vi "ai_continuous_and_ao_waveform_pc_infinite.vi"() -> ()   [LabVIEW 2020]
uses:
  <vilib>/measure/NI_MABase.lvlib
panel:
  out "error out 2":errorcluster caption="错误输出"
  in  "停止":bool
  out "Rounds 2":i32
  out "x-y":u32
  out "波形图 2":waveform(dbl)(graph)
  in  "SamplePeriod":u32=10000
  in  "Chan":u8
  out "Rounds":i32
  out "error out":errorcluster caption="错误输出"
  out "AiFifoResidual":i32
  in  "Stop":bool
  out "波形图":sgl[][](graph)
  in  "PointsToRead":u32=500
  in  "SamplePeriod(ns)":u32=20000
  in  "ChanSel":bool[](array[boolean])=[TRUE, TRUE, TRUE, TRUE, TRUE, TRUE, TRUE, TRUE, FALSE, FALSE, FALSE, FALSE, FALSE, FALSE, FALSE, FALSE, FALSE, FALSE, FALSE, FALSE, FALSE, FALSE, FALSE, FALSE]
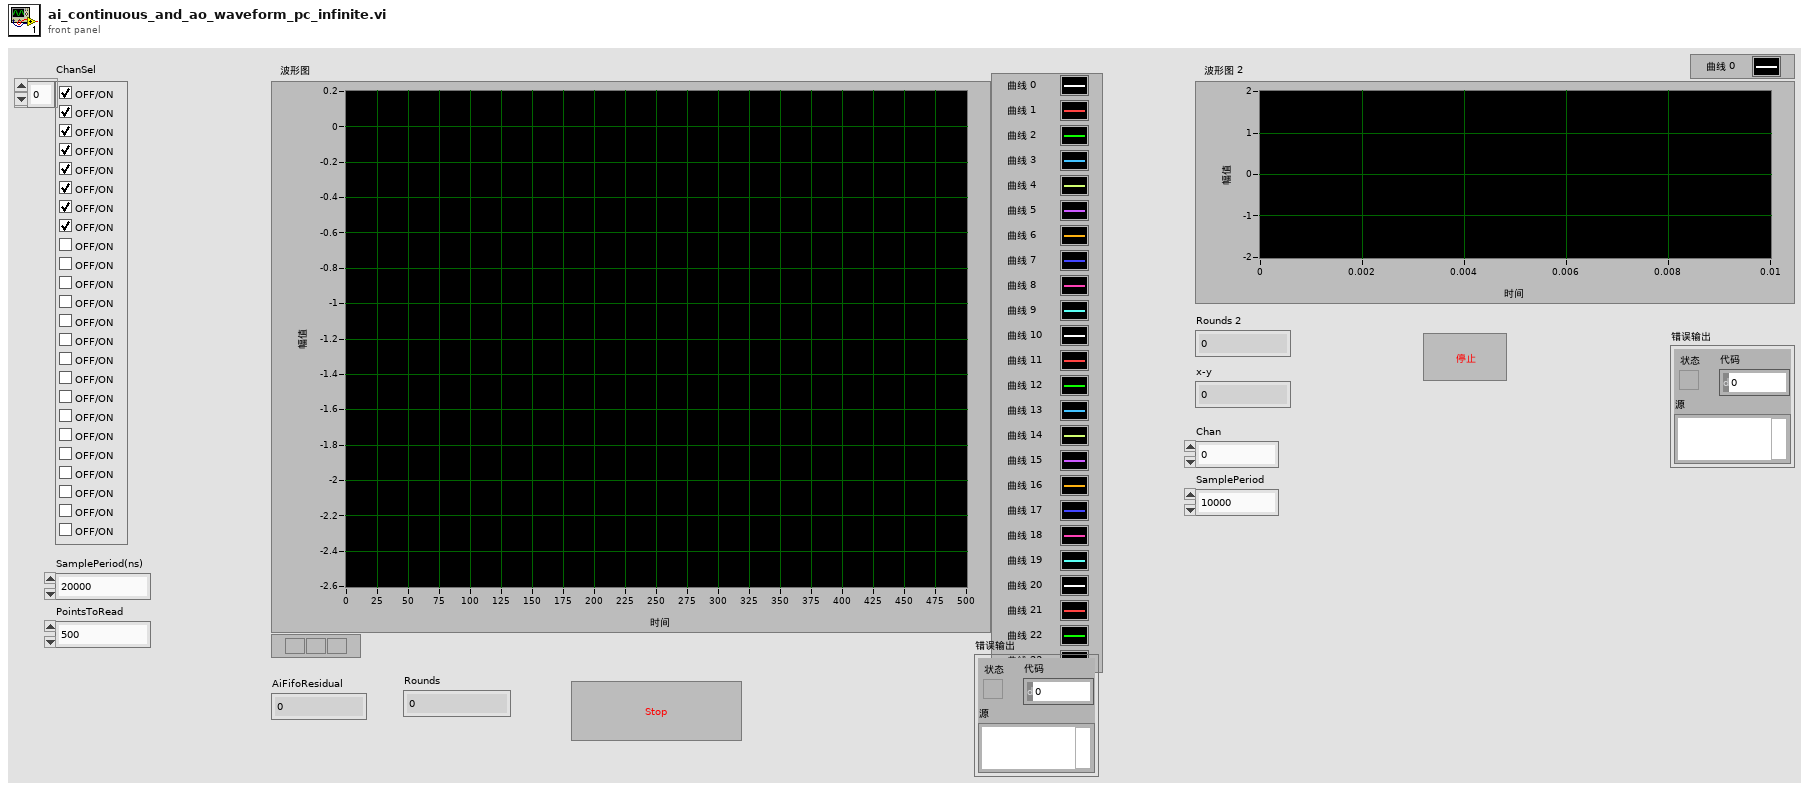
[diagram p1: front panel]
types:
  T1 = enum16{"Sine Wave", "Triangle Wave", "Square Wave", "Sawtooth Wave"}
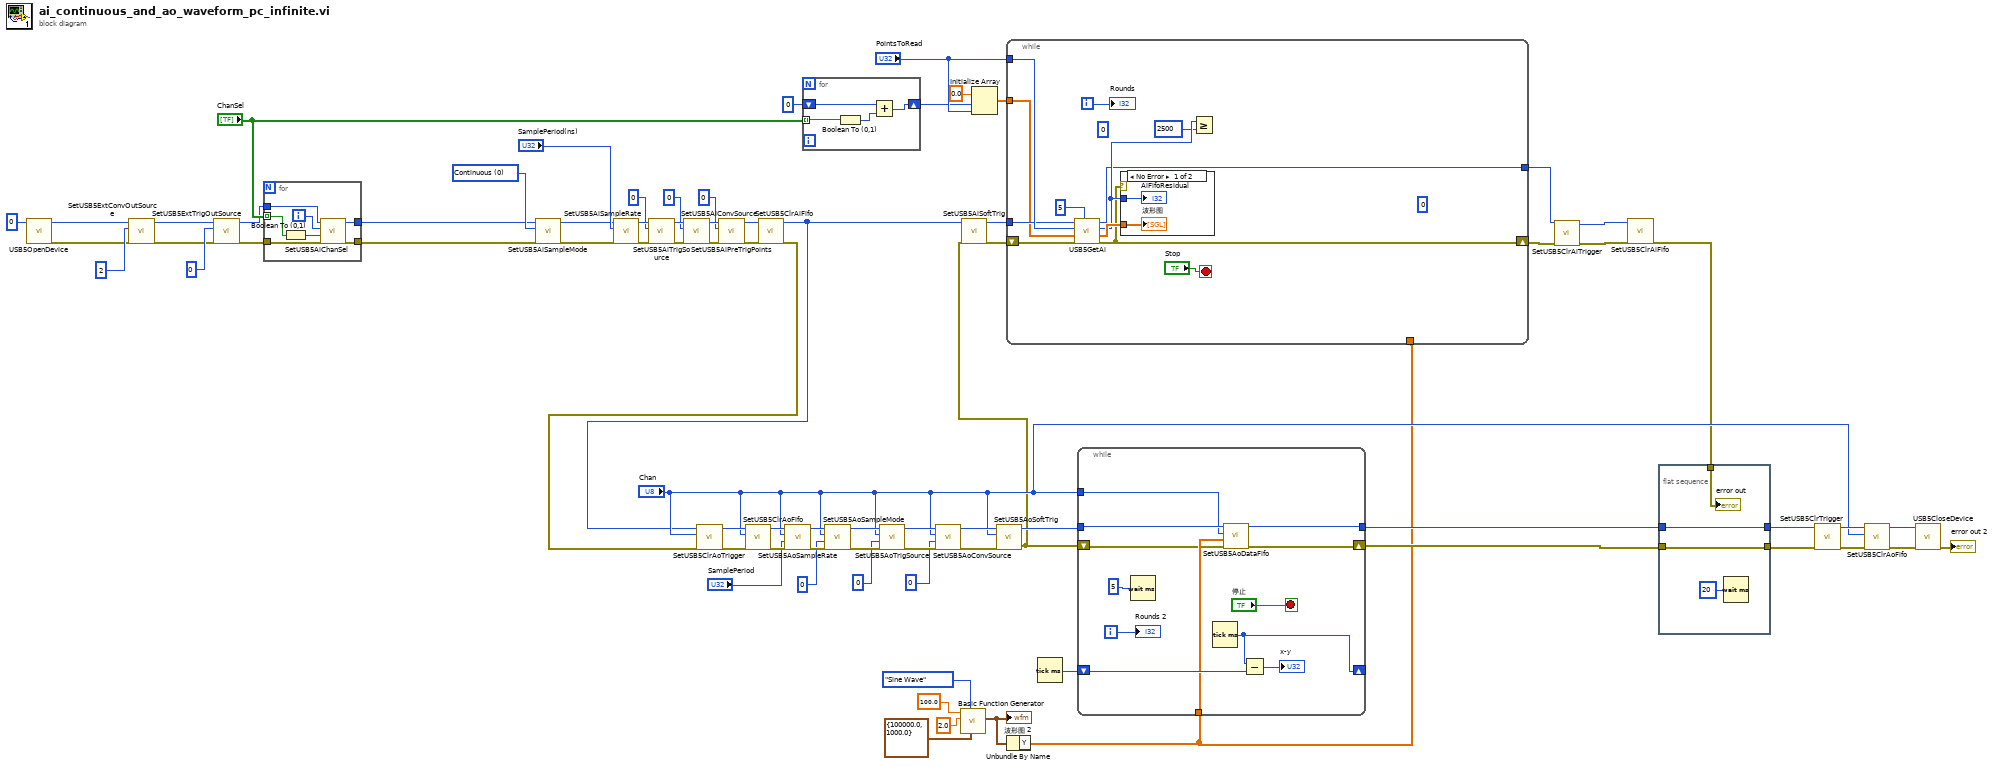
[diagram p0: block diagram]
diagram:
  w74 = u8 0 items=["Continuous", "OneShot"] ("AiSampleMode")
  n1 = call "USB5OpenDevice.vi"("DevIndex"=0) -> ("error out"=w48:errorcluster, "DevIndex Out"=w49:i32)  [unwired: 9 in]
  n2 = call "SetUSB5ExtConvOutSource.vi"("错误输入（无错误）"=w48, "Source"=u8 2, "DevIndex"=w49) -> ("错误输出"=w46:errorcluster, "DevIndex Out"=w47:i32)  [unwired: 7 in]
  n3 = call "SetUSB5ExtTrigOutSource.vi"("错误输入（无错误）"=w46, "Source"=u8 0, "DevIndex"=w47) -> ("错误输出"=w50:errorcluster, "DevIndex Out"=w51:i32)  [unwired: 7 in]
  n4 = for {
    tunnel: w51 -> [w83]
    tunnel: w50 -> [w82]
    tunnel: [w79] -> w4
    tunnel: [w78] -> w3
    tunnel: "ChanSel" -> [w77] mode=indexing
    i -> [w81]
    n5 = Boolean To (0,1)(Boolean=w77) -> (0, 1=w80:i16)
    n6 = call "SetUSB5AiChanSel.vi"("错误输入（无错误）"=w82, "Sel"=w80, "Chan"=w81, "DevIndex"=w83) -> ("错误输出"=w78:errorcluster, "DevIndex Out"=w79:i32)  [unwired: 6 in]
  }
  n7 = call "SetUSB5AiSampleMode.vi"("错误输入（无错误）"=w3, "AiSampleMode"=w74, "DevIndex"=w4) -> ("错误输出"=w5:errorcluster, "DevIndex Out"=w6:i32)  [unwired: 7 in]
  n8 = call "SetUSB5AiSampleRate.vi"("错误输入（无错误）"=w5, "SamplePeriod(ns)"="SamplePeriod(ns)", "DevIndex"=w6) -> ("错误输出"=w72:errorcluster, "DevIndex Out"=w73:i32)  [unwired: 7 in]
  n9 = call "SetUSB5AiTrigSource.vi"("错误输入（无错误）"=w72, "AiTrigSource"=u8 0, "DevIndex"=w73) -> ("错误输出"=w69:errorcluster, "DevIndex Out"=w70:i32)  [unwired: 7 in]
  n10 = call "SetUSB5AiConvSource.vi"("错误输入（无错误）"=w69, "AiConvSource"=u8 0, "DevIndex"=w70) -> ("错误输出"=w66:errorcluster, "DevIndex Out"=w67:i32)  [unwired: 7 in]
  n11 = call "SetUSB5AiPreTrigPoints.vi"("错误输入（无错误）"=w66, "AiPreTrigPoints"=u32 0, "DevIndex"=w67) -> ("错误输出"=w63:errorcluster, "DevIndex Out"=w64:i32)  [unwired: 7 in]
  n12 = call "SetUSB5ClrAiFifo.vi"("错误输入（无错误）"=w63, "DevIndex"=w64) -> ("错误输出"=w9:errorcluster, "DevIndex Out"=w13:i32)  [unwired: 8 in]
  n13 = call "SetUSB5ClrAoTrigger.vi"("错误输入（无错误）"=w9, "Chan"="Chan", "DevIndex"=w13) -> ("错误输出"=w38:errorcluster, "DevIndex Out"=w39:i32)  [unwired: 7 in]
  n14 = call "SetUSB5ClrAoFifo.vi"("错误输入（无错误）"=w38, "Chan"="Chan", "DevIndex"=w39) -> ("错误输出"=w45:errorcluster, "DevIndex Out"=w44:i32)  [unwired: 7 in]
  n15 = call "SetUSB5AoSampleRate.vi"("错误输入（无错误）"=w45, "SamplePeriod(ns)"="SamplePeriod", "Chan"="Chan", "DevIndex"=w44) -> ("错误输出"=w41:errorcluster, "DevIndex Out"=w42:i32)  [unwired: 6 in]
  n16 = for {
    tunnel: "ChanSel" -> [w87] mode=indexing
    shift-right: [w84] -> w55
    shift-left: i16 0 -> [w85]
    n17 = Boolean To (0,1)(Boolean=w87) -> (0, 1=w86:i16)
    n18 = Add(x=w85, y=w86) -> (x+y=w84:i16)
  }
  n19 = call "SetUSB5AoSampleMode.vi"("错误输入（无错误）"=w41, "SampleMode"=u8 0, "Chan"="Chan", "DevIndex"=w42) -> ("错误输出"=w36:errorcluster, "DevIndex Out"=w37:i32)  [unwired: 6 in]
  n20 = call "SetUSB5AoTrigSource.vi"("错误输入（无错误）"=w36, "AoTrigSource"=u8 0, "Chan"="Chan", "DevIndex"=w37) -> ("错误输出"=w34:errorcluster, "DevIndex Out"=w35:i32)  [unwired: 6 in]
  n21 = call "SetUSB5AoConvSource.vi"("错误输入（无错误）"=w34, "AoConvSource"=u8 0, "Chan"="Chan", "DevIndex"=w35) -> ("错误输出"=w32:errorcluster, "DevIndex Out"=w33:i32)  [unwired: 6 in]
  n22 = call <vilib>:"Basic Function Generator.vi"("sampling info"=cluster{"Fs":dbl, "#s":dbl} {"Fs"=100000.0, "#s"=1000.0}, "signal type"=T1."Sine Wave", "amplitude"=2.0, "frequency"=100.0) -> ("signal out"=w25:waveform(dbl))  [unwired: 5 in, 2 out]
  "波形图 2" <- w25
  n23 = Initialize Array(sgl 0.0 ("元素"), w55, "PointsToRead") -> (w57:sgl[][])
  n24 = call "SetUSB5AoSoftTrig.vi"("错误输入（无错误）"=w32, "Chan"="Chan", "DevIndex"=w33) -> ("错误输出"=w12:errorcluster, "DevIndex Out"=w15:i32)  [unwired: 7 in]
  n25 = call "SetUSB5AiSoftTrig.vi"("错误输入（无错误）"=w12, "DevIndex"=w13) -> ("错误输出"=w61:errorcluster, "DevIndex Out"=w62:i32)  [unwired: 8 in]
  n26 = Unbundle By Name(w25) -> ("Y"=w10:dbl[])
  n27 = while {
    tunnel: w62 -> [w92]
    tunnel: "PointsToRead" -> [w98]
    tunnel: w57 -> [w91]
    shift-right: [w88] -> w8
    shift-left: w61 -> [w99]
    tunnel: w10 -> [_]
    tunnel: [w89] -> w1
    i -> [w95]
    stop <- "Stop" stop-if-true
    (unwired) u8 0 ("Chan")
    (unwired) 0 ("禁用的索引 (列)")
    n28 = call "USB5GetAi.vi"("TimeOut"=5, "错误输入（无错误）"=w99, "Ai"=w91, "Points"=w98, "DevIndex"=w92) -> ("错误输出"=w88:errorcluster, "Ai Out"=w94:sgl[][], "AiFifoUsed"=w93:i32, "DevIndex Out"=w89:i32)  [unwired: 3 in]
    n29 = case shown="No Error" w88 {
      tunnel: w93 -> [w101 _]
      tunnel: w94 -> [w100 _]
      frame No Error {
        "波形图" <- w100
        "AiFifoResidual" <- w101
      }
      frame Error {
      }
    }
    n30 = Greater Or Equal?(x=w93, y=2500) -> ()  [unwired: 1 out]
    "Rounds" <- w95
  }
  n31 = Tick Count (ms)() -> (millisecond timer value=w16:u32)
  n32 = while {
    tunnel: w15 -> [w107]
    tunnel: "Chan" -> [w102]
    tunnel: w10 -> [w105]
    tunnel: [w106] -> w18
    shift-right: [w103] -> w17
    shift-left: w12 -> [w104]
    shift-right: [w109] -> _
    shift-left: w16 -> [w111]
    i -> [w112]
    stop <- "停止" stop-if-true
    n33 = Wait (ms)(milliseconds to wait=u32 5 ("毫秒倍数")) -> ()  [unwired: 1 out]
    n34 = Tick Count (ms)() -> (millisecond timer value=w109:u32)
    n35 = call "SetUSB5AoDataFifo.vi"("错误输入（无错误）"=w104, "Voltage"=w105, "Chan"=w102, "DevIndex"=w107) -> ("错误输出"=w103:errorcluster, "DevIndex Out"=w106:i32)  [unwired: 6 in]
    n36 = Subtract(x=w109, y=w111) -> (x-y=→"x-y":u32)
    "Rounds 2" <- w112
  }
  n37 = call "SetUSB5ClrAiTrigger.vi"("错误输入（无错误）"=w8, "DevIndex"=w1) -> ("错误输出"=w11:errorcluster, "DevIndex Out"=w54:i32)  [unwired: 8 in]
  n38 = call "SetUSB5ClrAiFifo.vi"("错误输入（无错误）"=w11, "DevIndex"=w54) -> ("错误输出"=w2:errorcluster)  [unwired: 8 in, 1 out]
  n39 = flat-sequence {
    tunnel: [w117] -> w19
    tunnel: w18 -> [w117]
    tunnel: w17 -> [w115]
    tunnel: [w115] -> w7
    tunnel: w2 -> [w114]
    frame #0 {
      n40 = Wait (ms)(milliseconds to wait=u32 20 ("等待时间（毫秒）")) -> ()  [unwired: 1 out]
      "error out" <- w114
    }
  }
  n41 = call "SetUSB5ClrTrigger.vi"("错误输入（无错误）"=w7, "DevIndex"=w19) -> ("错误输出"=w23:errorcluster, "DevIndex Out"=w24:i32)  [unwired: 8 in]
  n42 = call "SetUSB5ClrAoFifo.vi"("错误输入（无错误）"=w23, "Chan"="Chan", "DevIndex"=w24) -> ("错误输出"=w21:errorcluster, "DevIndex Out"=w22:i32)  [unwired: 7 in]
  n43 = call "USB5CloseDevice.vi"("错误输入（无错误）"=w21, "DevIndex"=w22) -> ("error out"=→"error out 2":errorcluster)  [unwired: 8 in, 1 out]
